vi "send_message.vi"(8 "error in (no error)":errorcluster, 10 "message":T1, 11 "StreamingBase in":refnum<class "StreamingBase.lvclass">) -> (0 "error out":errorcluster, 3 "StreamingBase out":refnum<class "StreamingBase.lvclass">)   [LabVIEW 2011, in "StreamingBase.lvclass"]
uses:
  StreamingBase.lvclass
  message_enum.ctl
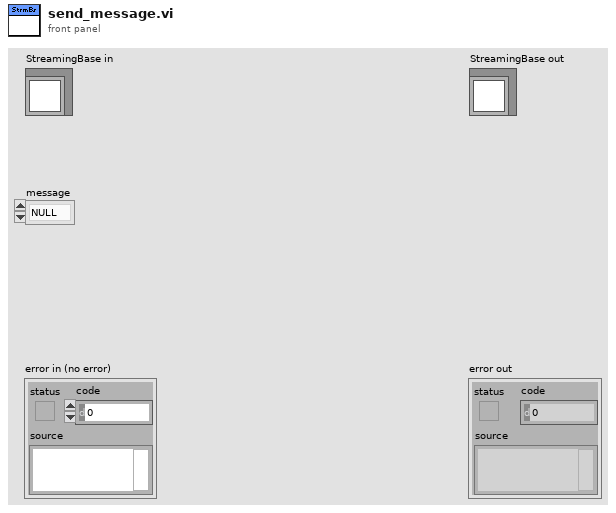
[diagram p1: front panel]
types:
  T1 = typedef "StreamingBase.lvclass/message_enum.ctl" = enum16{"NULL", "initialise", "terminate", "register as observer", "attach observer", "detach observer", "start", "stop"}
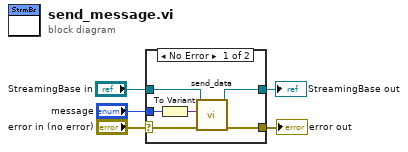
[diagram p0: block diagram]
diagram:
  n1 = case shown="No Error" "error in (no error)" {
    selector: "error in (no error)" -> [w10 w13]
    tunnel: [w9 w13] -> w4
    tunnel: [w6 w12] -> w2
    tunnel: "StreamingBase in" -> [w7 w12]
    tunnel: "message" -> [w11 _]
    frame No Error {
      n2 = To Variant(anything=w11) -> (Variant=w8:variant)
      n3 = call-dynamic "send_data.vi"("error in (no error)"=w10, "data variant"=w8, "StreamingBase in"=w7) -> ("error out"=w9:errorcluster, "StreamingBase out"=w6:refnum<class "StreamingBase.lvclass">)  [unwired: 7 in]
    }
    frame Error {
    }
  }
  "error out" <- w4
  "StreamingBase out" <- w2
